vi "PR4000 cfg slave enable.vi"(8 "error in (no error)":errorcluster, 10 "Channel parsed command info":T1, 11 "MKS4000b in":refnum<class "MKS4000b.lvclass">) -> (0 "error out":errorcluster, 2 "new commands":string, 3 "MKS4000b out":refnum<class "MKS4000b.lvclass">)   [LabVIEW 2020, in "MKS4000b.lvclass"]
uses:
  MKS4000b.lvclass
  channel parsed cmd cluster.ctl
  channel_mode_typdef.ctl
  MKS4000b.lvclass/MKS4000b.ctl
  CompressAndUpdate(Enum).vi
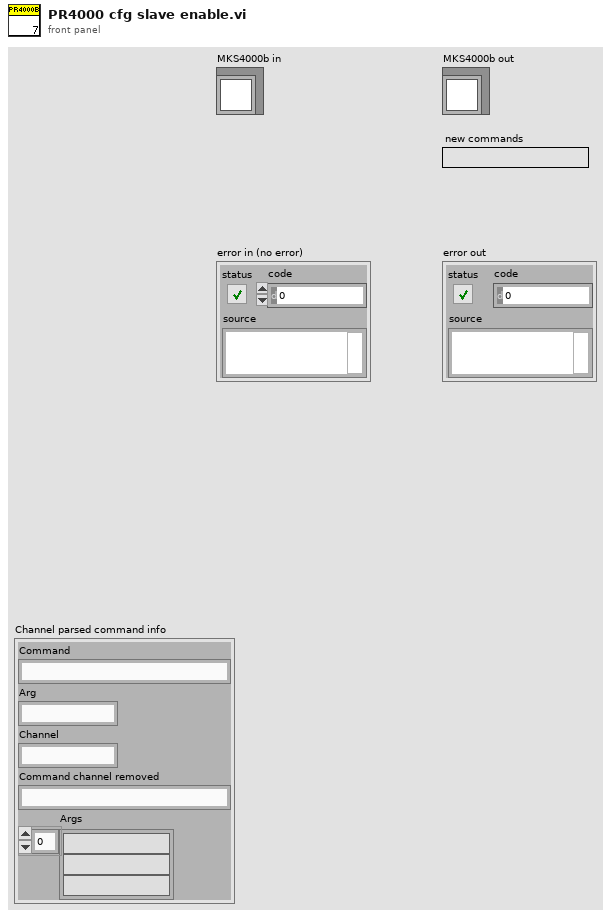
[diagram p1: front panel]
types:
  T1 = typedef "channel parsed cmd cluster.ctl" = cluster{"Command":string, "Arg":string, "Channel":string, "Command channel removed":string, "Args":string[]}
  T2 = typedef "channel_mode_typdef.ctl" = enum16{"Pressure", "Flow"}
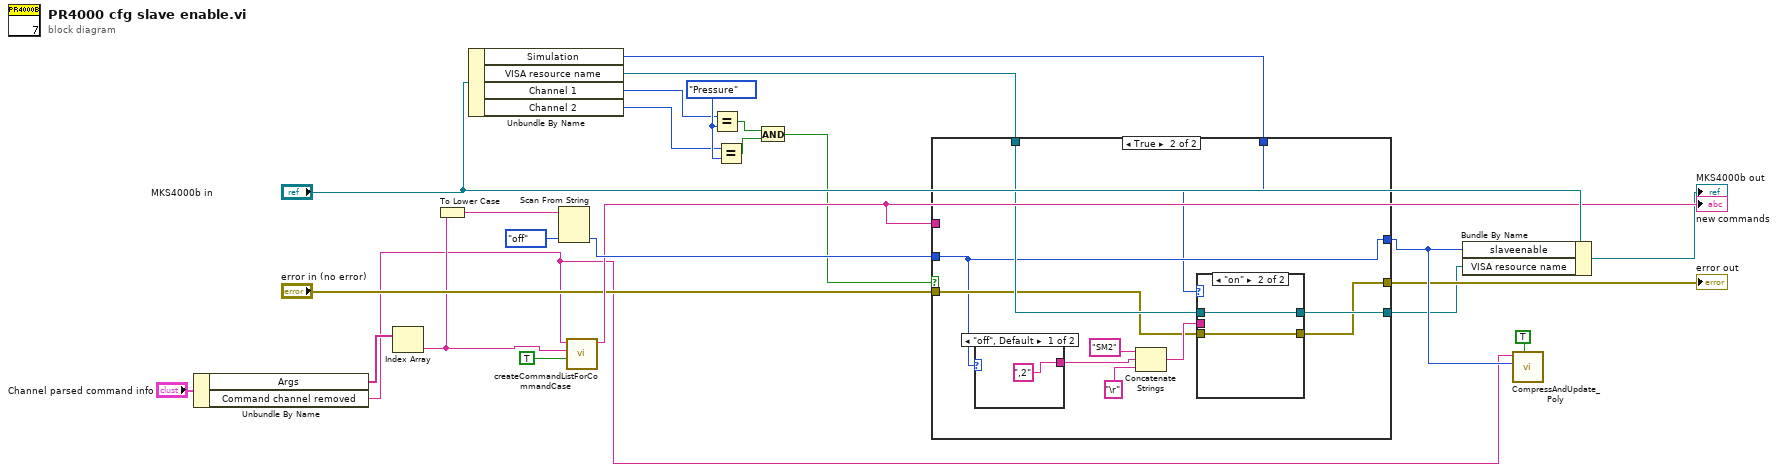
[diagram p0: block diagram]
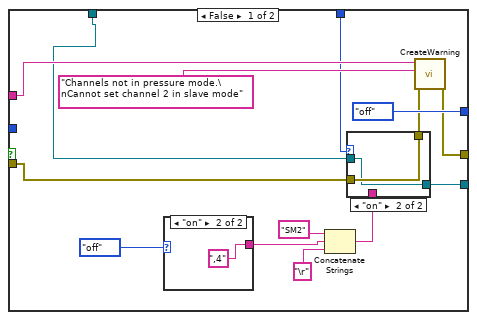
[diagram p2: hidden frame]
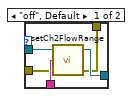
[diagram p3: hidden frame]
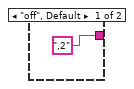
[diagram p4: hidden frame]
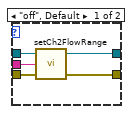
[diagram p5: hidden frame]
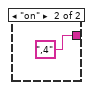
[diagram p6: hidden frame]
diagram:
  w15 = channel_mode_typdef."Pressure" ("Settings.Mode.Channel 1")
  n1 = Unbundle By Name("Channel parsed command info") -> ("Args"=w2:string[], "Command channel removed"=w1:string)
  n2 = Index Array(array=w2) -> (element=w8:string)  [unwired: 1 in]
  n3 = To Lower Case(string=w8) -> (all lower case string=w7:string)
  n4 = Unbundle By Name("MKS4000b in") -> ("Simulation"=w24:enum16{"off", "on"}, "VISA resource name"=w9:refnum<visa-resource-name>, "Channel 1"=w13:T2, "Channel 2"=w14:T2)
  n5 = Scan From String(input string=w7, default 1=enum16{"off", "on"}."off" ("Settings.Save")) -> (output 1=w20:enum16{"off", "on"})  [unwired: 3 in, 3 out]
  n6 = call "createCommandListForCommandCase.vi"("immediate Check (only once)"=TRUE, "setvalue"=w8, "command"=w1) -> ("new commands"=w19:string)  [unwired: 8 in]
  "new commands" <- w19
  n7 = Equal?(x=w13, y=w15) -> (x = y?=w16:bool)
  n8 = Equal?(x=w14, y=w15) -> (x = y?=w17:bool)
  n9 = And(x=w16, y=w17) -> (x .and. y?=w18:bool)
  n10 = case shown="True" w18 {
    tunnel: w9 -> [w30 w57]
    tunnel: [w29 w56] -> w10
    tunnel: "error in (no error)" -> [w28 w53]
    tunnel: [w26 w52] -> w12
    tunnel: w19 -> [w38 _]
    tunnel: w20 -> [_ w49]
    tunnel: [enum16{"off", "on"}."off" ("Settings.Save") w49] -> w23
    tunnel: w24 -> [w25 w48]
    frame False {
      n11 = case shown="\"on\"" enum16{"off", "on"}."off" ("Settings.Save") {
        tunnel: [",2" ("string") ",4" ("string")] -> w32
        frame "off", Default {
        }
        frame "on" {
        }
      }
      n12 = Concatenate Strings("SM2" ("string"), w32, "\r" ("string")) -> (w34:string)
      n13 = case shown="\"on\"" w25 {
        tunnel: w34 -> [w43 _]
        tunnel: w30 -> [w42 w44]
        tunnel: [w41 w44] -> w29
        tunnel: w28 -> [w40 w45]
        tunnel: [w39 w45] -> w27
        frame "off", Default {
          n14 = call "setCh2FlowRange.vi"("error"=w40, "command in"=w43, "Comport PR4000"=w42) -> ("error out"=w39:errorcluster, "VISA resource name out"=w41:refnum<visa-resource-name>)  [unwired: 1 out]
        }
        frame "on" {
        }
      }
      n15 = call "CreateWarning.vi"("user error in"=w27, "error message (\"\")"="Channels not in pressure mode.\nCannot set channel 2 in slave mode" ("error message (\"\")"), "command"=w38) -> ("user error  out"=w26:errorcluster)  [unwired: 8 in]
    }
    frame True {
      n16 = case shown="\"off\", Default" w49 {
        tunnel: [",2" ("string") ",4" ("string")] -> w50
        frame "off", Default {
        }
        frame "on" {
        }
      }
      n17 = Concatenate Strings("SM2" ("string"), w50, "\r" ("string")) -> (w54:string)
      n18 = case shown="\"on\"" w48 {
        tunnel: w57 -> [w62 w64]
        tunnel: [w61 w64] -> w56
        tunnel: w54 -> [w60 _]
        tunnel: w53 -> [w59 w63]
        tunnel: [w58 w63] -> w52
        frame "off", Default {
          n19 = call "setCh2FlowRange.vi"("error"=w59, "command in"=w60, "Comport PR4000"=w62) -> ("error out"=w58:errorcluster, "VISA resource name out"=w61:refnum<visa-resource-name>)  [unwired: 1 out]
        }
        frame "on" {
        }
      }
    }
  }
  "error out" <- w12
  n20 = Bundle By Name(cluster="MKS4000b in", "slaveenable"=w23, "VISA resource name"=w10) -> (→"MKS4000b out":refnum<class "MKS4000b.lvclass">)
  n21 = call-poly "CompressAndUpdate_Poly.vi"("force CVT update (false)"=TRUE ("force CVT update"), "enum variant"=w23, "command or variable name"=w1) -> ()  [unwired: 8 in, 1 out]
